vi "Get_Do.vi"(0 "reference in":refnum<class "Sig_DO_Simple.lvclass">) -> (8 "DO":bool)   [LabVIEW 2019, in "Sig_DO_Simple.lvclass"]
uses:
  Sig_DO_Simple.lvclass
  Sig_DO_Simple.lvclass/Sig_DO_Simple.ctl
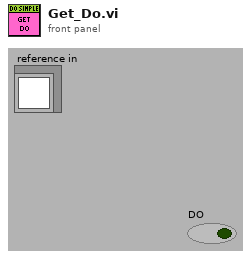
[diagram p1: front panel]
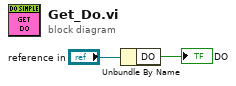
[diagram p0: block diagram]
diagram:
  n1 = Unbundle By Name("reference in") -> ("DO"=→"DO":bool)
